vi "Engr_interface.vi"() -> ()   [LabVIEW 2016]
uses:
  Type_Defs/Digital_Out.ctl
  Type_Defs/Digital_In_1.ctl
  Type_Defs/Analog_In.ctl
  <vilib>/httpClient/ClientHandle.ctl
  msg7171_linux.llb/send single message.vi
  <vilib>/httpClient/POSTBuffer.vi
  <vilib>/httpClient/LabVIEWHTTPClient.lvlib
panel:
  out "Analog in":T1
  in  "LN2 Platen":u16(slide) max=4095 step=1 scale=0.0..4095.0
  in  "LN2 Shroud":u16(slide) max=4095 step=1 scale=0.0..4095.0
  out "Digi_In_1":T2
  in  "Digi_Out":T3
  in  "Regen Standby Mode SP":u8 max=1 step=1
  in  "Regen Repurge Time SP":u16=5 max=9999 step=1
  in  "Pumps per Compressor SP":u8=1 min=1 max=3 step=1
  in  "Regen Rough Interlock SP":u8=1 max=1 step=1
  in  "Regen Restart Temp SP":u8 max=80 step=1
  in  "Regen Rt of Rise Cycles SP":u8=50 max=200 step=1
  in  "Regen Rate of Rise SP":u8=10 min=1 max=100 step=1
  in  "Regen Rough to Press SP":u8=100 min=25 max=200 step=1
  in  "Regen Repurge Cycles SP":u8=50 max=200 step=1
  in  "Regen Ext Purge Time SP":u16 max=9990 step=1
  in  "MCC_2sgTempCtl":u16 max=320 step=1
  out "MCC_1sgTempCtll V":string
  out "MCC_2sgTempCtl V":string
  out "Regen Restart Delay":string
  in  "1st Ctl type":u8(ring) items=["ExtHeat", "1st s ctl", "2nd sctl", "Dual"]
  out "MCC_RegenCycles":string
  out "CryoP OP Time":string
  out "MCC_Status":string
  in  "Log?":bool
  out "Resp":string
  out "MCC Pwr":bool
  out "MCC Error":bool
  out "MCC_TurnTcOn_V":string
  out "MCC_TurnRoughOn_V":string
  out "MCC_TurnPurgeOn_V":string
  in  "MCC_StartRegen_V":u8(ring) items=["Abort Regen", "Start Full", "Start Fast", "Exit Standby", "Warm&Stop"]
  out "MCC 2nd stage Temp":string
  out "1st stage Temp":string
  out "MCCget_Ver_V":string
  out "MCC_RoughInterlock_V":string
  out "MCC_RegenSeq":string
  out "Regen Standby Mode":string
  out "Regen Repurge Time":string
  out "Pumps per Compressor":string
  out "Regen Rough Interlock":string
  out "Regen Restart Temp":string
  out "Regen Rt of Rise Cycles":string
  out "Regen Rate of Rise":string
  out "Regen Rough to Press":string
  out "Regen Repurge Cycles":string
  out "Regen Ext Purge Time":string
  in  "Regen Restart Delay SP":u16 max=59994 step=1
  out "DutyCycle":string
  out "MCC_TCpres":string
  in  "Get MCC":bool
  out "MCC_RegenTime":string
  in  "MCC_clearRoughInterlock":bool
  out "MCC_RegenError":string
  in  "MCC_StartRegen":bool
  in  "MCC_TurnTcOn":bool
  in  "MCC_OpenRoughGateValve":bool
  in  "MCC_OpenPurgeValve":bool
  in  "MCC_TurnPumpOn":bool
  in  "MCC_1sgTempCtl":u16 max=320 step=1
  in  "Params":bool
  in  "Get DIO":bool=TRUE
  in  "Get PG":bool
  out "x/y":T4 {"Rouffing Pump" format="%#_6e"; "Chamber Pressure" format="%#_6e"; "Cryo Pump" format="%#_6e"}
  in  "exit":bool
  out "Waveform Chart":waveform(dbl)[](graph)=[{"t0"=timestamp(3580757854.087 s since 1904-01-01), "dt"=1.0, "Y"=[750.0616827041697]}, {"t0"=timestamp(3580757854.087 s since 1904-01-01), "dt"=1.0, "Y"=[750.0616827041697]}, {"t0"=timestamp(3580757854.087 s since 1904-01-01), "dt"=1.0, "Y"=[750.0616827041697]}]
  out "MCC_PumpState":string
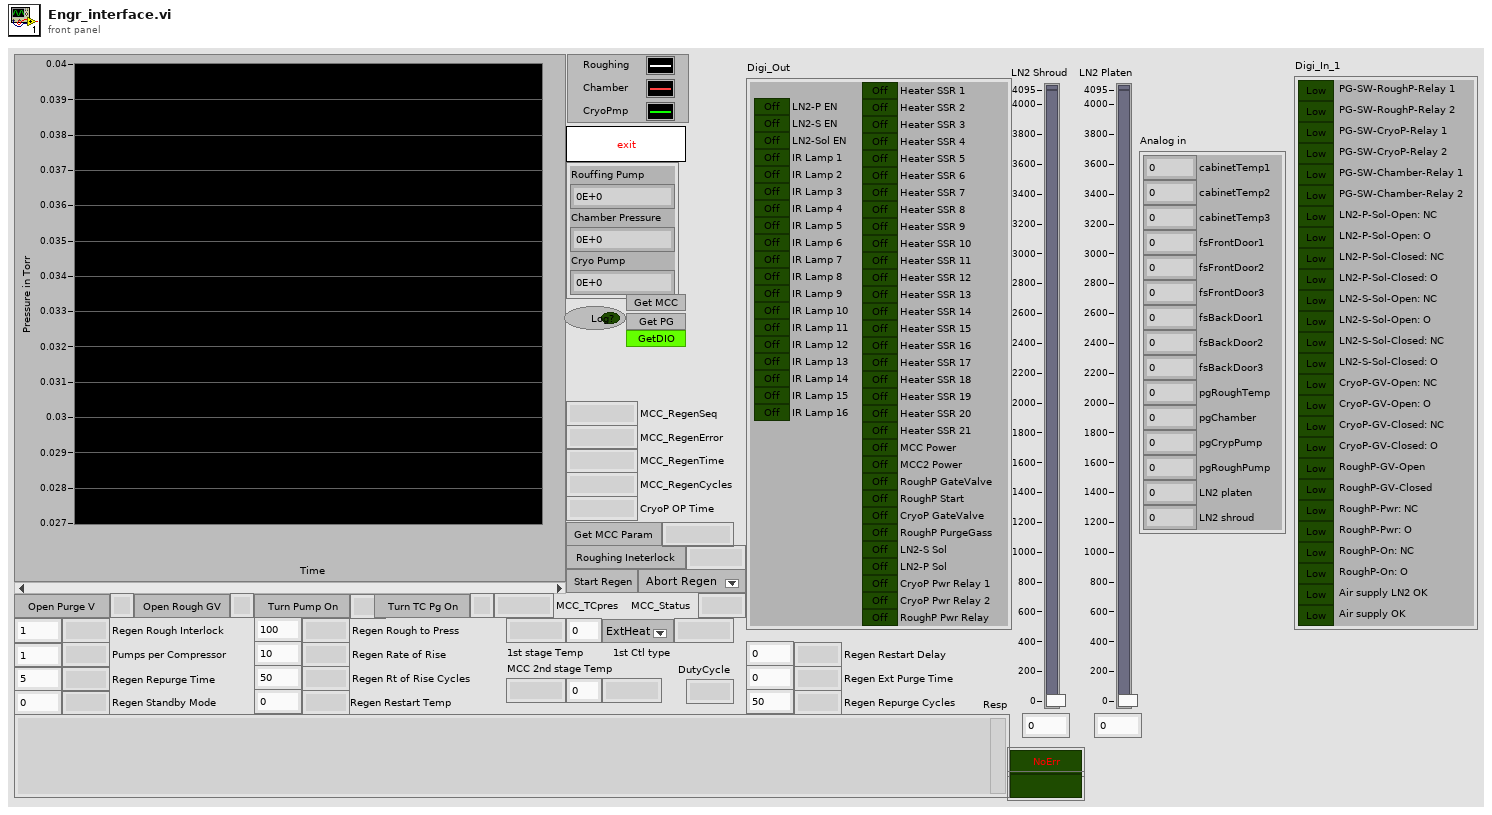
[diagram p1: front panel]
types:
  T1 = typedef "Analog_In.ctl" = cluster{"cabinetTemp1":u16, "cabinetTemp2":u16, "cabinetTemp3":u16, "fsFrontDoor1":u16, "fsFrontDoor2":u16, "fsFrontDoor3":u16, "fsBackDoor1":u16, "fsBackDoor2":u16, "fsBackDoor3":u16, "pgRoughTemp":u16, "pgChamber":u16, "pgCrypPump":u16, "pgRoughPump":u16, "LN2 platen":u16, "LN2 shroud":u16}
  T2 = typedef "Digital_In_1.ctl" = cluster{"PG-SW-RoughP-Relay 1":bool, "PG-SW-RoughP-Relay 2":bool, "PG-SW-CryoP-Relay 1":bool, "PG-SW-CryoP-Relay 2":bool, "PG-SW-Chamber-Relay 1":bool, "PG-SW-Chamber-Relay 2":bool, "LN2-P-Sol-Open: NC":bool, "LN2-P-Sol-Open: O":bool, "LN2-P-Sol-Closed: NC":bool, "LN2-P-Sol-Closed: O":bool, "LN2-S-Sol-Open: NC":bool, "LN2-S-Sol-Open: O":bool, "LN2-S-Sol-Closed: NC":bool, "LN2-S-Sol-Closed: O":bool, "CryoP-GV-Open: NC":bool, "CryoP-GV-Open: O":bool, "CryoP-GV-Closed: NC":bool, "CryoP-GV-Closed: O":bool, "RoughP-GV-Open":bool, "RoughP-GV-Closed":bool, "RoughP-Pwr: NC":bool, "RoughP-Pwr: O":bool, "RoughP-On: NC":bool, "RoughP-On: O":bool, "Air supply LN2 OK":bool, "Air supply OK":bool}
  T3 = typedef "Digital_Out.ctl" = cluster{"LN2-P EN":bool, "LN2-S EN":bool, "LN2-Sol EN":bool, "IR Lamp 1":bool, "IR Lamp 2":bool, "IR Lamp 3":bool, "IR Lamp 4":bool, "IR Lamp 5":bool, "IR Lamp 6":bool, "IR Lamp 7":bool, "IR Lamp 8":bool, "IR Lamp 9":bool, "IR Lamp 10":bool, "IR Lamp 11":bool, "IR Lamp 12":bool, "IR Lamp 13":bool, "IR Lamp 14":bool, "IR Lamp 15":bool, "IR Lamp 16":bool, "Heater SSR 1":bool, "Heater SSR 2":bool, "Heater SSR 3":bool, "Heater SSR 4":bool, "Heater SSR 5":bool, "Heater SSR 6":bool, "Heater SSR 7":bool, "Heater SSR 8":bool, "Heater SSR 9":bool, "Heater SSR 10":bool, "Heater SSR 11":bool, "Heater SSR 12":bool, "Heater SSR 13":bool, "Heater SSR 14":bool, "Heater SSR 15":bool, "Heater SSR 16":bool, "Heater SSR 17":bool, "Heater SSR 18":bool, "Heater SSR 19":bool, "Heater SSR 20":bool, "Heater SSR 21":bool, "MCC Power":bool, "MCC2 Power":bool, "RoughP GateValve":bool, "RoughP Start":bool, "CryoP GateValve":bool, "RoughP PurgeGass":bool, "LN2-S Sol":bool, "LN2-P Sol":bool, "CryoP Pwr Relay 1":bool, "CryoP Pwr Relay 2":bool, "RoughP Pwr Relay":bool}
  T4 = cluster{"Rouffing Pump":dbl, "Chamber Pressure":dbl, "Cryo Pump":dbl}
  T5 = typedef "LabVIEWHTTPClient.lvlib/ClientHandle.ctl" = refnum<k1>
  T6 = cluster{"go":bool, "Http session":T5, "URL prefex":string}
  T7 = cluster{"Addr":i32[], "Kind":string[], "Pressure":dbl[], "Sw1 SP":dbl[], "Sw2 SP":dbl[]}
  T8 = cluster{"Error":bool, "PowerFailure":bool, "Data":string}
  T9 = cluster{"Status":string, "TcPressure":string, "TempStage1":string, "TempStage2":string, "Duty Cycle":string, "RegenStep":string, "RegenError":string, "CryoPumpRdyState":string}
  T10 = cluster{"MCCVersion":string, "ElapsedTime":string, "FirstStageTempCTL":string, "PurgeValveState":string, "RegenCycles":string, "RegenParam_0":string, "RegenParam_1":string, "RegenParam_2":string, "RegenParam_3":string, "RegenParam_4":string, "RegenParam_5":string, "RegenParam_6":string, "RegenParam_A":string, "RegenParam_C":string, "RegenParam_G":string, "RegenParam_z":string, "RegenTime":string, "RoughingValveState":string, "RoughingInterlock":string, "SecondStageTempCTL":string, "TcPressureState":string}
  T11 = cluster{"event":string, "event":string, "JSON string":string}
  T12 = cluster{"event":string, "event":string, "event":string}
  T13 = cluster{"Pressure[0]":dbl, "Pressure[1]":dbl, "Pressure[2]":dbl}
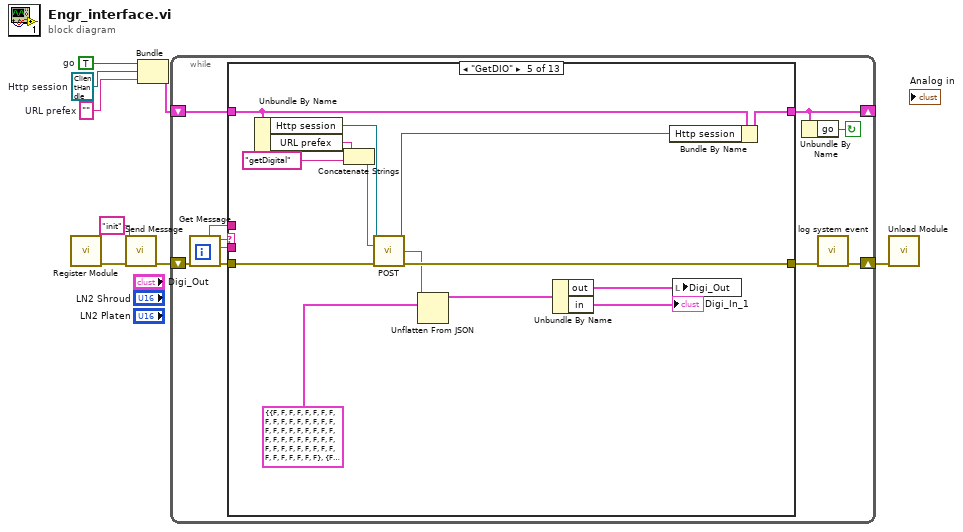
[diagram p0: block diagram]
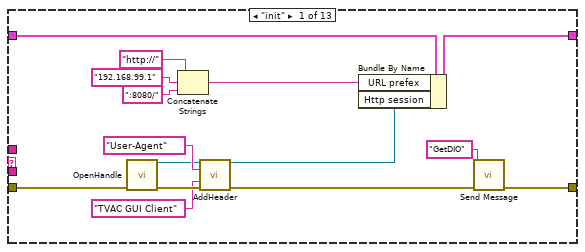
[diagram p2: hidden frame]
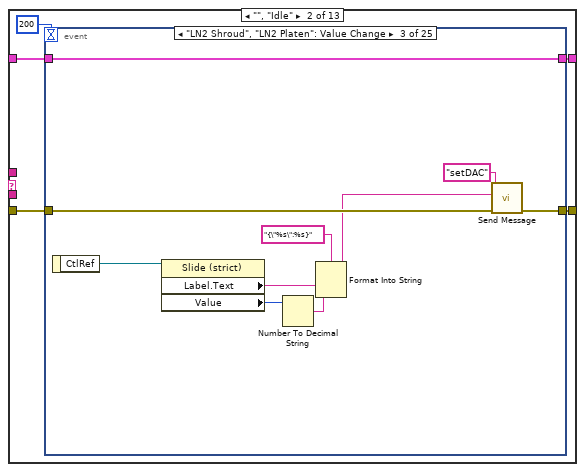
[diagram p3: hidden frame]
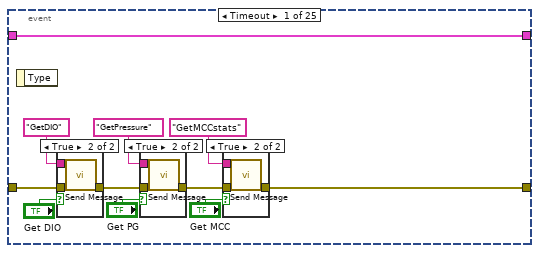
[diagram p4: hidden frame]
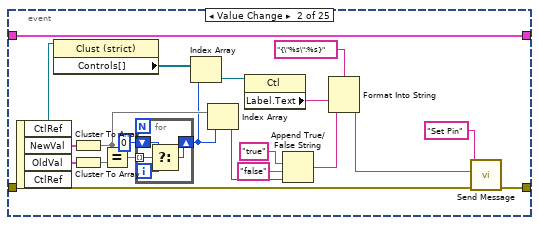
[diagram p8: hidden frame]
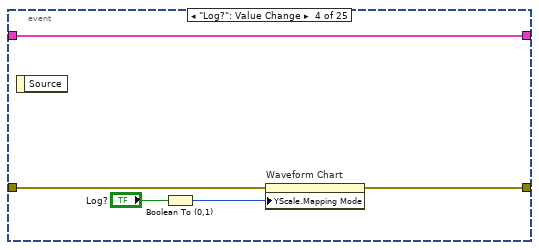
[diagram p9: hidden frame]
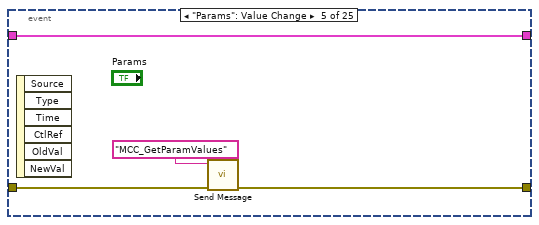
[diagram p10: hidden frame]
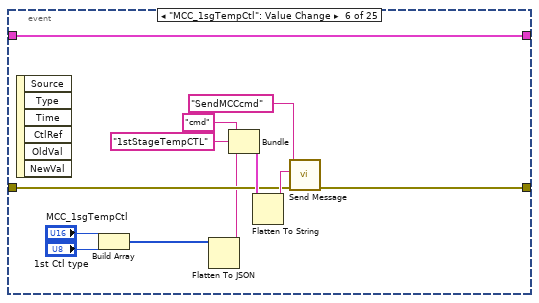
[diagram p11: hidden frame]
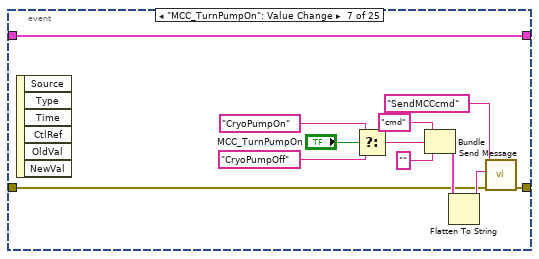
[diagram p12: hidden frame]
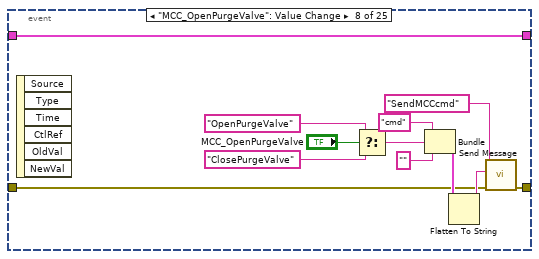
[diagram p13: hidden frame]
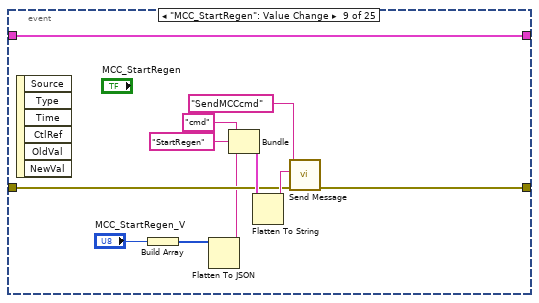
[diagram p14: hidden frame]
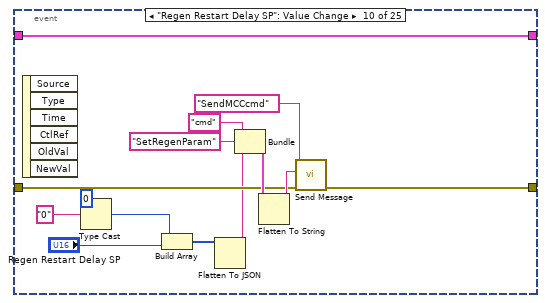
[diagram p15: hidden frame]
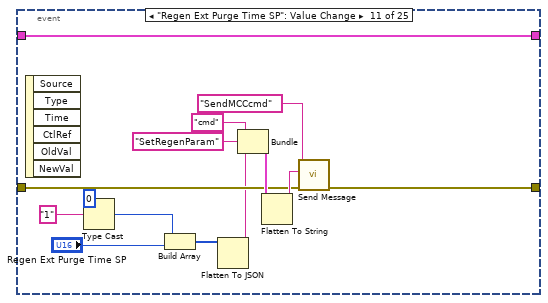
[diagram p16: hidden frame]
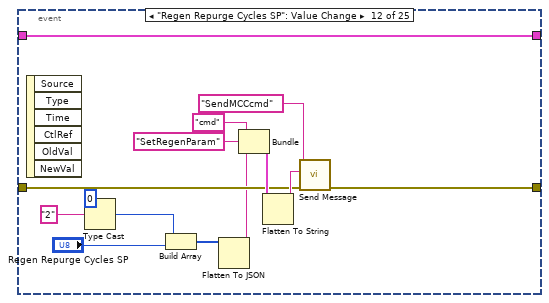
[diagram p17: hidden frame]
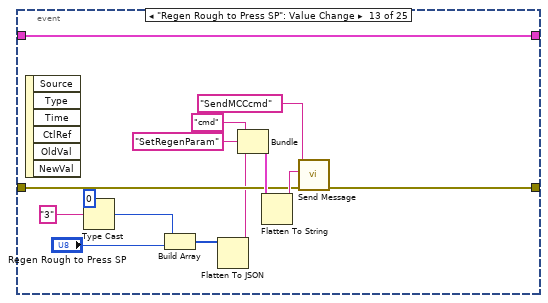
[diagram p18: hidden frame]
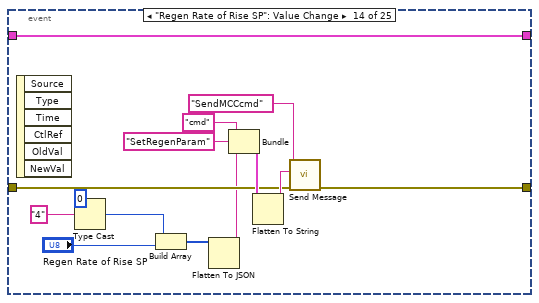
[diagram p19: hidden frame]
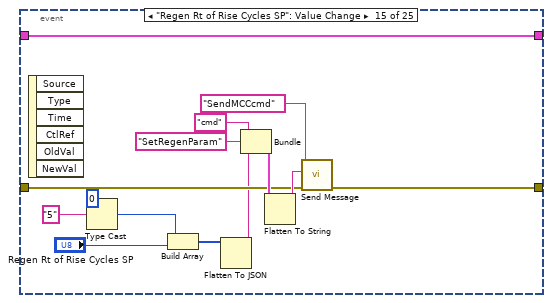
[diagram p20: hidden frame]
diagram:
  w4 = ""  # URL prefex
  w5 = T5 refnum  # Http session
  w6 = TRUE  # go
  n1 = call "Register Module.vi"() -> ("error out"=w2:errorcluster)  [unwired: 10 in, 1 out]
  n2 = call-poly "Send Message.vi"("error in (no error)"=w2, "event"="init") -> ("error out"=w1:errorcluster)  [unwired: 9 in]
  n3 = Bundle("go"=w6, "Http session"=w5, "URL prefex"=w4) -> (w8:T6)  [unwired: 1 in]
  n4 = while {
    shift-left: w8 -> [w15]
    shift-right: [w12] -> _
    shift-right: [w10] -> w7
    shift-left: w1 -> [w18]
    stop <- w11 continue-if-true
    n5 = call "Get Message.vi"("error in (no error)"=w18) -> ("error out"=w16:errorcluster, "event buffer"=w17:string, "event"=w14:string, "source"=w13:string)  [unwired: 7 in]
    n6 = case shown="\"GetDIO\"" w14 {
      selector: w14 -> [_ _ w360 _ _ _ _ _ _ _ _ _ w540]
      tunnel: [w24 w35 w364 w386 w398 w418 w447 w456 w473 w504 w531 w537 w542] -> w12
      tunnel: w15 -> [w33 w34 w363 w385 w397 w416 w447 w456 w471 w504 w531 w532 w542]
      tunnel: w17 -> [_ _ w358 w382 _ _ _ _ w465 w502 w529 _ _]
      tunnel: w16 -> [w28 w36 w362 w384 w400 w420 w440 w449 w474 w505 w530 w535 w541]
      tunnel: w13 -> [_ _ _ _ _ _ _ _ _ _ _ _ w539]
      tunnel: [w20 w38 w361 w383 w399 w419 w439 w448 w459 w505 w530 w534 w538] -> w9
      frame "init" {
        n7 = call <vilib>:"OpenHandle.vi"("error in (no error)"=w28) -> ("client handle out"=w29:T5, "error out"=w32:errorcluster)  [unwired: 13 in]
        n8 = Concatenate Strings("http://" ("url"), "192.168.99.1" ("Address"), ":8080/" ("url")) -> (w23:string)
        n9 = call <vilib>:"AddHeader.vi"("client handle"=w29, "header"="User-Agent", "value"="TVAC GUI Client", "error in (no error)"=w32) -> ("client handle out"=w22:T5, "error out"=w21:errorcluster)  [unwired: 10 in]
        n10 = Bundle By Name(cluster=w33, "URL prefex"=w23, "Http session"=w22) -> (w24:T6)
        n11 = call-poly "Send Message.vi"("error in (no error)"=w21, "event"="GetDIO") -> ("error out"=w20:errorcluster)  [unwired: 9 in]
      }
      frame "", "Idle" {
        n12 = event shown="[2] \"LN2 Shroud\", \"LN2 Platen\": Value Change" {
          selector: _ -> [_ _ _ _ _ _ _ _ _ _ _ _ _ _ _ _ _ _ _ _ _ _ _ _ _]
          dyn-events: _ -> [_ _ _ _ _ _ _ _ _ _ _ _ _ _ _ _ _ _ _ _ _ _ _ _ _]
          timeout: 200 ("milliseconds to wait") -> [_ _ _ _ _ _ _ _ _ _ _ _ _ _ _ _ _ _ _ _ _ _ _ _ _]
          tunnel: w36 -> [w48 w77 w94 w100 w104 w111 w123 w135 w146 w160 w174 w188 w202 w216 w230 w244 w258 w272 w286 w300 w312 w322 w332 w344 w354]
          tunnel: [w39 w76 w95 w99 w103 w110 w122 w134 w145 w159 w173 w187 w201 w215 w229 w243 w257 w271 w285 w299 w311 w321 w331 w343 w353] -> w38
          tunnel: [w49 w82 w87 w101 w102 w112 w124 w136 w147 w161 w175 w189 w203 w217 w231 w245 w259 w273 w287 w301 w313 w323 w333 w345 w351] -> w35
          tunnel: w34 -> [w49 w82 w87 w101 w102 w112 w124 w136 w147 w161 w175 w189 w203 w217 w231 w245 w259 w273 w287 w301 w313 w323 w333 w345 w351]
          event Timeout {
            n13 = event-data() -> ()  [unwired: 1 in, 1 out]
            n14 = case shown="True" "Get DIO" {
              tunnel: w48 -> [w58 w61]
              tunnel: [w58 w60] -> w46
              tunnel: "GetDIO" ("event") -> [_ w59]
              frame False {
              }
              frame True {
                n15 = call-poly "Send Message.vi"("error in (no error)"=w61, "event"=w59) -> ("error out"=w60:errorcluster)  [unwired: 9 in]
              }
            }
            n16 = case shown="True" "Get PG" {
              tunnel: w46 -> [w54 w57]
              tunnel: [w54 w56] -> w40
              tunnel: "GetPressure" ("event") -> [_ w55]
              frame False {
              }
              frame True {
                n17 = call-poly "Send Message.vi"("error in (no error)"=w57, "event"=w55) -> ("error out"=w56:errorcluster)  [unwired: 9 in]
              }
            }
            n18 = case shown="True" "Get MCC" {
              tunnel: w40 -> [w50 w53]
              tunnel: [w50 w52] -> w39
              tunnel: "GetMCCstats" ("event") -> [_ w51]
              frame False {
              }
              frame True {
                n19 = call-poly "Send Message.vi"("error in (no error)"=w53, "event"=w51) -> ("error out"=w52:errorcluster)  [unwired: 9 in]
              }
            }
          }
          event Value Change {
            n20 = event-data() -> ("CtlRef"=w63:refnum<vi>, "NewVal"=w78:T3, "OldVal"=w81:T3)  [unwired: 1 in, 1 out]
            n21 = property class="Clust (strict)"(reference=w63) -> ("Controls[]"=w73:refnum<vi>[])  [unwired: 1 in, 2 out]
            n22 = Cluster To Array(cluster=w78) -> (array=w74:bool[])
            n23 = Cluster To Array(cluster=w81) -> (array=w75:bool[])
            n24 = Equal?(x=w74, y=w75) -> (x = y?=w80:bool[])
            n25 = for {
              tunnel: w80 -> [w86] mode=indexing
              shift-right: [w85] -> w72
              shift-left: 0 -> [w84]
              i -> [w83]
              n26 = Select(t=w84, s=w86, f=w83) -> (s? t:f=w85:i32)
            }
            n27 = Index Array(array=w73, index=w72) -> (element=w71:refnum<vi>)
            n28 = Index Array(array=w74, index=w72) -> (element=w69:bool)
            n29 = property class="Ctl"(reference=w71) -> ("Label.Text"=w66:string)  [unwired: 1 in, 2 out]
            n30 = Append True/False String(1:w69, 2:"false" ("false string"), 3:"true" ("true string")) -> (0:w64:string)  [unwired: 1 in]
            n31 = Format Into String(format string="{\"%s\":%s}" ("string"), w66, w64) -> (resulting string=w62:string)  [unwired: 2 in, 1 out]
            n32 = call-poly "Send Message.vi"("error in (no error)"=w77, "event buffer"=w62, "event"="Set Pin") -> ("error out"=w76:errorcluster)  [unwired: 8 in]
          }
          event "LN2 Shroud", "LN2 Platen": Value Change {
            n33 = event-data() -> ("CtlRef"=w93:refnum<vi>)  [unwired: 1 in]
            n34 = property class="Slide (strict)"(reference=w93) -> ("Label.Text"=w91:string, "Value"=w90:u16)  [unwired: 1 in, 2 out]
            n35 = Number To Decimal String(number=w90) -> (decimal integer string=w89:string)  [unwired: 1 in]
            n36 = Format Into String(format string="{\"%s\":%s}" ("string"), w91, w89) -> (resulting string=w88:string)  [unwired: 2 in, 1 out]
            n37 = call-poly "Send Message.vi"("error in (no error)"=w94, "event buffer"=w88, "event"="setDAC") -> ("error out"=w95:errorcluster)  [unwired: 8 in]
          }
          event "Log?": Value Change {
            n38 = event-data() -> ()  [unwired: 1 in, 1 out]
            n39 = Boolean To (0,1)(Boolean="Log?") -> (0, 1=w98:i16)
            n40 = property on="Waveform Chart" class="WFChart (strict)"(error in=w100, "YScale.Mapping Mode"=w98) -> (error out=w99:errorcluster)  [unwired: 1 in, 1 out]
          }
          event "Params": Value Change {
            n41 = event-data() -> ()  [unwired: 1 in, 6 out]
            n42 = call-poly "Send Message.vi"("error in (no error)"=w104, "event"="MCC_GetParamValues") -> ("error out"=w103:errorcluster)  [unwired: 9 in]
          }
          event "MCC_1sgTempCtl": Value Change {
            n43 = event-data() -> ()  [unwired: 1 in, 6 out]
            n44 = Build Array("MCC_1sgTempCtl", "1st Ctl type") -> (w107:u16[])
            n45 = Flatten To JSON(anything=w107) -> (JSON string=w106:string)  [unwired: 2 in, 1 out]
            n46 = Bundle("event"="cmd", "event"="1stStageTempCTL", "JSON string"=w106) -> (w115:T11)  [unwired: 1 in]
            n47 = Flatten To String(anything=w115) -> (data string=w116:string)  [unwired: 3 in, 2 out]
            n48 = call-poly "Send Message.vi"("error in (no error)"=w111, "event buffer"=w116, "event"="SendMCCcmd") -> ("error out"=w110:errorcluster)  [unwired: 8 in]
          }
          event "MCC_TurnPumpOn": Value Change {
            n49 = event-data() -> ()  [unwired: 1 in, 6 out]
            n50 = Select(t="CryoPumpOn" ("event"), s="MCC_TurnPumpOn", f="CryoPumpOff" ("event")) -> (s? t:f=w120:string)
            n51 = Bundle("event"="cmd", "event"=w120, "event"="") -> (w127:T12)  [unwired: 1 in]
            n52 = Flatten To String(anything=w127) -> (data string=w128:string)  [unwired: 3 in, 2 out]
            n53 = call-poly "Send Message.vi"("error in (no error)"=w123, "event buffer"=w128, "event"="SendMCCcmd") -> ("error out"=w122:errorcluster)  [unwired: 8 in]
          }
          event "MCC_OpenPurgeValve": Value Change {
            n54 = event-data() -> ()  [unwired: 1 in, 6 out]
            n55 = Select(t="OpenPurgeValve" ("event"), s="MCC_OpenPurgeValve", f="ClosePurgeValve" ("event")) -> (s? t:f=w132:string)
            n56 = Bundle("event"="cmd", "event"=w132, "event"="") -> (w139:T12)  [unwired: 1 in]
            n57 = Flatten To String(anything=w139) -> (data string=w140:string)  [unwired: 3 in, 2 out]
            n58 = call-poly "Send Message.vi"("error in (no error)"=w135, "event buffer"=w140, "event"="SendMCCcmd") -> ("error out"=w134:errorcluster)  [unwired: 8 in]
          }
          event "MCC_StartRegen": Value Change {
            n59 = event-data() -> ()  [unwired: 1 in, 6 out]
            n60 = Build Array("MCC_StartRegen_V") -> (w143:u8[])
            n61 = Flatten To JSON(anything=w143) -> (JSON string=w144:string)  [unwired: 2 in, 1 out]
            n62 = Bundle("event"="cmd", "event"="StartRegen", "JSON string"=w144) -> (w150:T11)  [unwired: 1 in]
            n63 = Flatten To String(anything=w150) -> (data string=w151:string)  [unwired: 3 in, 2 out]
            n64 = call-poly "Send Message.vi"("error in (no error)"=w146, "event buffer"=w151, "event"="SendMCCcmd") -> ("error out"=w145:errorcluster)  [unwired: 8 in]
          }
          event "Regen Restart Delay SP": Value Change {
            n65 = event-data() -> ()  [unwired: 1 in, 6 out]
            n66 = Type Cast(type=u8 0 ("unsigned 8bit integer"), x="0") -> (*(type *) &x=w154:u8)
            n67 = Build Array(w154, "Regen Restart Delay SP") -> (w158:u16[])
            n68 = Flatten To JSON(anything=w158) -> (JSON string=w157:string)  [unwired: 2 in, 1 out]
            n69 = Bundle("event"="cmd", "event"="SetRegenParam", "JSON string"=w157) -> (w164:T11)  [unwired: 1 in]
            n70 = Flatten To String(anything=w164) -> (data string=w165:string)  [unwired: 3 in, 2 out]
            n71 = call-poly "Send Message.vi"("error in (no error)"=w160, "event buffer"=w165, "event"="SendMCCcmd") -> ("error out"=w159:errorcluster)  [unwired: 8 in]
          }
          event "Regen Ext Purge Time SP": Value Change {
            n72 = event-data() -> ()  [unwired: 1 in, 6 out]
            n73 = Type Cast(type=u8 0 ("unsigned 8bit integer"), x="1") -> (*(type *) &x=w168:u8)
            n74 = Build Array(w168, "Regen Ext Purge Time SP") -> (w172:u16[])
            n75 = Flatten To JSON(anything=w172) -> (JSON string=w171:string)  [unwired: 2 in, 1 out]
            n76 = Bundle("event"="cmd", "event"="SetRegenParam", "JSON string"=w171) -> (w178:T11)  [unwired: 1 in]
            n77 = Flatten To String(anything=w178) -> (data string=w179:string)  [unwired: 3 in, 2 out]
            n78 = call-poly "Send Message.vi"("error in (no error)"=w174, "event buffer"=w179, "event"="SendMCCcmd") -> ("error out"=w173:errorcluster)  [unwired: 8 in]
          }
          event "Regen Repurge Cycles SP": Value Change {
            n79 = event-data() -> ()  [unwired: 1 in, 6 out]
            n80 = Type Cast(type=u8 0 ("unsigned 8bit integer"), x="2") -> (*(type *) &x=w182:u8)
            n81 = Build Array(w182, "Regen Repurge Cycles SP") -> (w186:u8[])
            n82 = Flatten To JSON(anything=w186) -> (JSON string=w185:string)  [unwired: 2 in, 1 out]
            n83 = Bundle("event"="cmd", "event"="SetRegenParam", "JSON string"=w185) -> (w192:T11)  [unwired: 1 in]
            n84 = Flatten To String(anything=w192) -> (data string=w193:string)  [unwired: 3 in, 2 out]
            n85 = call-poly "Send Message.vi"("error in (no error)"=w188, "event buffer"=w193, "event"="SendMCCcmd") -> ("error out"=w187:errorcluster)  [unwired: 8 in]
          }
          event "Regen Rough to Press SP": Value Change {
            n86 = event-data() -> ()  [unwired: 1 in, 6 out]
            n87 = Type Cast(type=u8 0 ("unsigned 8bit integer"), x="3") -> (*(type *) &x=w196:u8)
            n88 = Build Array(w196, "Regen Rough to Press SP") -> (w200:u8[])
            n89 = Flatten To JSON(anything=w200) -> (JSON string=w199:string)  [unwired: 2 in, 1 out]
            n90 = Bundle("event"="cmd", "event"="SetRegenParam", "JSON string"=w199) -> (w206:T11)  [unwired: 1 in]
            n91 = Flatten To String(anything=w206) -> (data string=w207:string)  [unwired: 3 in, 2 out]
            n92 = call-poly "Send Message.vi"("error in (no error)"=w202, "event buffer"=w207, "event"="SendMCCcmd") -> ("error out"=w201:errorcluster)  [unwired: 8 in]
          }
          event "Regen Rate of Rise SP": Value Change {
            n93 = event-data() -> ()  [unwired: 1 in, 6 out]
            n94 = Type Cast(type=u8 0 ("unsigned 8bit integer"), x="4") -> (*(type *) &x=w210:u8)
            n95 = Build Array(w210, "Regen Rate of Rise SP") -> (w214:u8[])
            n96 = Flatten To JSON(anything=w214) -> (JSON string=w213:string)  [unwired: 2 in, 1 out]
            n97 = Bundle("event"="cmd", "event"="SetRegenParam", "JSON string"=w213) -> (w220:T11)  [unwired: 1 in]
            n98 = Flatten To String(anything=w220) -> (data string=w221:string)  [unwired: 3 in, 2 out]
            n99 = call-poly "Send Message.vi"("error in (no error)"=w216, "event buffer"=w221, "event"="SendMCCcmd") -> ("error out"=w215:errorcluster)  [unwired: 8 in]
          }
          event "Regen Rt of Rise Cycles SP": Value Change {
            n100 = event-data() -> ()  [unwired: 1 in, 6 out]
            n101 = Type Cast(type=u8 0 ("unsigned 8bit integer"), x="5") -> (*(type *) &x=w224:u8)
            n102 = Build Array(w224, "Regen Rt of Rise Cycles SP") -> (w228:u8[])
            n103 = Flatten To JSON(anything=w228) -> (JSON string=w227:string)  [unwired: 2 in, 1 out]
            n104 = Bundle("event"="cmd", "event"="SetRegenParam", "JSON string"=w227) -> (w234:T11)  [unwired: 1 in]
            n105 = Flatten To String(anything=w234) -> (data string=w235:string)  [unwired: 3 in, 2 out]
            n106 = call-poly "Send Message.vi"("error in (no error)"=w230, "event buffer"=w235, "event"="SendMCCcmd") -> ("error out"=w229:errorcluster)  [unwired: 8 in]
          }
          event "Regen Restart Temp SP": Value Change {
            n107 = event-data() -> ()  [unwired: 1 in, 6 out]
            n108 = Type Cast(type=u8 0 ("unsigned 8bit integer"), x="6") -> (*(type *) &x=w238:u8)
            n109 = Build Array(w238, "Regen Restart Temp SP") -> (w242:u8[])
            n110 = Flatten To JSON(anything=w242) -> (JSON string=w241:string)  [unwired: 2 in, 1 out]
            n111 = Bundle("event"="cmd", "event"="SetRegenParam", "JSON string"=w241) -> (w248:T11)  [unwired: 1 in]
            n112 = Flatten To String(anything=w248) -> (data string=w249:string)  [unwired: 3 in, 2 out]
            n113 = call-poly "Send Message.vi"("error in (no error)"=w244, "event buffer"=w249, "event"="SendMCCcmd") -> ("error out"=w243:errorcluster)  [unwired: 8 in]
          }
          event "Regen Rough Interlock SP": Value Change {
            n114 = event-data() -> ()  [unwired: 1 in, 6 out]
            n115 = Type Cast(type=u8 0 ("unsigned 8bit integer"), x="A") -> (*(type *) &x=w252:u8)
            n116 = Build Array(w252, "Regen Rough Interlock SP") -> (w256:u8[])
            n117 = Flatten To JSON(anything=w256) -> (JSON string=w255:string)  [unwired: 2 in, 1 out]
            n118 = Bundle("event"="cmd", "event"="SetRegenParam", "JSON string"=w255) -> (w262:T11)  [unwired: 1 in]
            n119 = Flatten To String(anything=w262) -> (data string=w263:string)  [unwired: 3 in, 2 out]
            n120 = call-poly "Send Message.vi"("error in (no error)"=w258, "event buffer"=w263, "event"="SendMCCcmd") -> ("error out"=w257:errorcluster)  [unwired: 8 in]
          }
          event "Pumps per Compressor SP": Value Change {
            n121 = event-data() -> ()  [unwired: 1 in, 6 out]
            n122 = Type Cast(type=u8 0 ("unsigned 8bit integer"), x="C") -> (*(type *) &x=w266:u8)
            n123 = Build Array(w266, "Pumps per Compressor SP") -> (w270:u8[])
            n124 = Flatten To JSON(anything=w270) -> (JSON string=w269:string)  [unwired: 2 in, 1 out]
            n125 = Bundle("event"="cmd", "event"="SetRegenParam", "JSON string"=w269) -> (w276:T11)  [unwired: 1 in]
            n126 = Flatten To String(anything=w276) -> (data string=w277:string)  [unwired: 3 in, 2 out]
            n127 = call-poly "Send Message.vi"("error in (no error)"=w272, "event buffer"=w277, "event"="SendMCCcmd") -> ("error out"=w271:errorcluster)  [unwired: 8 in]
          }
          event "Regen Repurge Time SP": Value Change {
            n128 = event-data() -> ()  [unwired: 1 in, 6 out]
            n129 = Type Cast(type=u8 0 ("unsigned 8bit integer"), x="G") -> (*(type *) &x=w280:u8)
            n130 = Build Array(w280, "Regen Repurge Time SP") -> (w284:u16[])
            n131 = Flatten To JSON(anything=w284) -> (JSON string=w283:string)  [unwired: 2 in, 1 out]
            n132 = Bundle("event"="cmd", "event"="SetRegenParam", "JSON string"=w283) -> (w290:T11)  [unwired: 1 in]
            n133 = Flatten To String(anything=w290) -> (data string=w291:string)  [unwired: 3 in, 2 out]
            n134 = call-poly "Send Message.vi"("error in (no error)"=w286, "event buffer"=w291, "event"="SendMCCcmd") -> ("error out"=w285:errorcluster)  [unwired: 8 in]
          }
          event "Regen Standby Mode SP": Value Change {
            n135 = event-data() -> ()  [unwired: 1 in, 6 out]
            n136 = Type Cast(type=u8 0 ("unsigned 8bit integer"), x="z") -> (*(type *) &x=w294:u8)
            n137 = Build Array(w294, "Regen Standby Mode SP") -> (w298:u8[])
            n138 = Flatten To JSON(anything=w298) -> (JSON string=w297:string)  [unwired: 2 in, 1 out]
            n139 = Bundle("event"="cmd", "event"="SetRegenParam", "JSON string"=w297) -> (w304:T11)  [unwired: 1 in]
            n140 = Flatten To String(anything=w304) -> (data string=w305:string)  [unwired: 3 in, 2 out]
            n141 = call-poly "Send Message.vi"("error in (no error)"=w300, "event buffer"=w305, "event"="SendMCCcmd") -> ("error out"=w299:errorcluster)  [unwired: 8 in]
          }
          event "MCC_OpenRoughGateValve": Value Change {
            n142 = event-data() -> ()  [unwired: 1 in, 6 out]
            n143 = Select(t="OpenRoughValve" ("event"), s="MCC_OpenRoughGateValve", f="CloseRoughValve" ("event")) -> (s? t:f=w309:string)
            n144 = Bundle("event"="cmd", "event"=w309, "event"="") -> (w316:T12)  [unwired: 1 in]
            n145 = Flatten To String(anything=w316) -> (data string=w317:string)  [unwired: 3 in, 2 out]
            n146 = call-poly "Send Message.vi"("error in (no error)"=w312, "event buffer"=w317, "event"="SendMCCcmd") -> ("error out"=w311:errorcluster)  [unwired: 8 in]
          }
          event "MCC_clearRoughInterlock": Value Change {
            n147 = event-data() -> ()  [unwired: 1 in, 6 out]
            n148 = Bundle("event"="cmd", "event"="ClearInterlock", "event"="") -> (w325:T12)  [unwired: 1 in]
            n149 = Flatten To String(anything=w325) -> (data string=w326:string)  [unwired: 3 in, 2 out]
            n150 = call-poly "Send Message.vi"("error in (no error)"=w322, "event buffer"=w326, "event"="SendMCCcmd") -> ("error out"=w321:errorcluster)  [unwired: 8 in]
          }
          event "MCC_2sgTempCtl": Value Change {
            n151 = event-data() -> ()  [unwired: 1 in, 6 out]
            n152 = Build Array("MCC_2sgTempCtl") -> (w328:u16[])
            n153 = Flatten To JSON(anything=w328) -> (JSON string=w330:string)  [unwired: 2 in, 1 out]
            n154 = Bundle("event"="cmd", "event"="2ndStageTempCTL", "JSON string"=w330) -> (w336:T11)  [unwired: 1 in]
            n155 = Flatten To String(anything=w336) -> (data string=w337:string)  [unwired: 3 in, 2 out]
            n156 = call-poly "Send Message.vi"("error in (no error)"=w332, "event buffer"=w337, "event"="SendMCCcmd") -> ("error out"=w331:errorcluster)  [unwired: 8 in]
          }
          event "MCC_TurnTcOn": Value Change {
            n157 = event-data() -> ()  [unwired: 1 in, 6 out]
            n158 = Select(t="TurnTcPresOn" ("event"), s="MCC_TurnTcOn", f="TurnTcPresOff" ("event")) -> (s? t:f=w341:string)
            n159 = Bundle("event"="cmd", "event"=w341, "event"="") -> (w348:T12)  [unwired: 1 in]
            n160 = Flatten To String(anything=w348) -> (data string=w349:string)  [unwired: 3 in, 2 out]
            n161 = call-poly "Send Message.vi"("error in (no error)"=w344, "event buffer"=w349, "event"="SendMCCcmd") -> ("error out"=w343:errorcluster)  [unwired: 8 in]
          }
          event "exit": Value Change {
            n162 = event-data() -> ()  [unwired: 1 in, 1 out]
            n163 = call "Deliver Message.vi"("error in (no error)"=w354, "event"="exit") -> ("error out"=w353:errorcluster)  [unwired: 9 in]
          }
        }
      }
      frame "Set Pin" {
        (unwired) "{\"RoughP Start\":true}" ("string")
        n164 = Unbundle By Name(w363) -> ("Http session"=w368:T5, "URL prefex"=w366:string)
        n165 = Concatenate Strings(w366, "setDigital" ("url")) -> (w367:string)
        n166 = call-poly <vilib>:"POST.vi"("client handle"=w368, "url"=w367, "buffer"=w358, "error in (no error)"=w362) -> ("client handle out"=w369:T5, "error out"=w359:errorcluster)  [unwired: 8 in, 2 out]
        n167 = Build Array(0) -> (w356:i32[])
        n168 = case shown="False" FALSE {
          tunnel: [w370 w381] -> w361
          tunnel: w360 -> [_ w380]
          tunnel: w359 -> [w370 w379]
          tunnel: w356 -> [_ w376]
          frame False {
          }
          frame True {
            n169 = Replace Array Subset(array=w376, new element=0 ("new element/subarray"), index=2) -> (w372:i32[])
            n170 = call-poly "Send Message.vi"("error in (no error)"=w379, "event"="GetDIO") -> ("error out"=w378:errorcluster)  [unwired: 9 in]
            n171 = Flatten To JSON(anything=w372) -> (JSON string=w373:string)  [unwired: 2 in, 1 out]
            n172 = Wait (ms)(milliseconds to wait=u32 50) -> ()  [unwired: 1 out]
            n173 = call-poly "Send Message.vi"("error in (no error)"=w378, "event buffer"=w373, "event"=w380) -> ("error out"=w381:errorcluster)  [unwired: 8 in]
          }
        }
        n174 = Bundle By Name(cluster=w363, "Http session"=w369) -> (w364:T6)
      }
      frame "setDAC" {
        n175 = Unbundle By Name(w385) -> ("Http session"=w390:T5, "URL prefex"=w388:string)
        n176 = Concatenate Strings(w388, "setAnalog" ("url")) -> (w389:string)
        n177 = call-poly <vilib>:"POST.vi"("client handle"=w390, "url"=w389, "buffer"=w382, "error in (no error)"=w384) -> ("client handle out"=w391:T5, "error out"=w383:errorcluster)  [unwired: 8 in, 2 out]
        n178 = Bundle By Name(cluster=w385, "Http session"=w391) -> (w386:T6)
      }
      frame "GetDIO" {
        n179 = Unbundle By Name(w397) -> ("Http session"=w404:T5, "URL prefex"=w402:string)
        n180 = Concatenate Strings(w402, "getDigital" ("url")) -> (w403:string)
        n181 = call-poly <vilib>:"POST.vi"("client handle"=w404, "url"=w403, "error in (no error)"=w400) -> ("client handle out"=w405:T5, "body"=w396:string, "error out"=w399:errorcluster)  [unwired: 9 in, 1 out]
        n182 = Unflatten From JSON(JSON string=w396, type and defaults=cluster{"out":T3, "in":T2} {"out"={"LN2-P EN"=FALSE, "LN2-S EN"=FALSE, "LN2-Sol EN"=FALSE, "IR Lamp 1"=FALSE, "IR Lamp 2"=FALSE, "IR Lamp 3"=FALSE, "IR Lamp 4"=FALSE, "IR Lamp 5"=FALSE, "IR Lamp 6"=FALSE, "IR Lamp 7"=FALSE, "IR Lamp 8"=FALSE, "IR Lamp 9"=FALSE, "IR Lamp 10"=FALSE, "IR Lamp 11"=FALSE, "IR Lamp 12"=FALSE, "IR Lamp 13"=FALSE, "IR Lamp 14"=FALSE, "IR Lamp 15"=FALSE, "IR Lamp 16"=FALSE, "Heater SSR 1"=FALSE, "Heater SSR 2"=FALSE, "Heater SSR 3"=FALSE, "Heater SSR 4"=FALSE, "Heater SSR 5"=FALSE, "Heater SSR 6"=FALSE, "Heater SSR 7"=FALSE, "Heater SSR 8"=FALSE, "Heater SSR 9"=FALSE, "Heater SSR 10"=FALSE, "Heater SSR 11"=FALSE, "Heater SSR 12"=FALSE, "Heater SSR 13"=FALSE, "Heater SSR 14"=FALSE, "Heater SSR 15"=FALSE, "Heater SSR 16"=FALSE, "Heater SSR 17"=FALSE, "Heater SSR 18"=FALSE, "Heater SSR 19"=FALSE, "Heater SSR 20"=FALSE, "Heater SSR 21"=FALSE, "MCC Power"=FALSE, "MCC2 Power"=FALSE, "RoughP GateValve"=FALSE, "RoughP Start"=FALSE, "CryoP GateValve"=FALSE, "RoughP PurgeGass"=FALSE, "LN2-S Sol"=FALSE, "LN2-P Sol"=FALSE, "CryoP Pwr Relay 1"=FALSE, "CryoP Pwr Relay 2"=FALSE, "RoughP Pwr Relay"=FALSE}, "in"={"PG-SW-RoughP-Relay 1"=FALSE, "PG-SW-RoughP-Relay 2"=FALSE, "PG-SW-CryoP-Relay 1"=FALSE, "PG-SW-CryoP-Relay 2"=FALSE, "PG-SW-Chamber-Relay 1"=FALSE, "PG-SW-Chamber-Relay 2"=FALSE, "LN2-P-Sol-Open: NC"=FALSE, "LN2-P-Sol-Open: O"=FALSE, "LN2-P-Sol-Closed: NC"=FALSE, "LN2-P-Sol-Closed: O"=FALSE, "LN2-S-Sol-Open: NC"=FALSE, "LN2-S-Sol-Open: O"=FALSE, "LN2-S-Sol-Closed: NC"=FALSE, "LN2-S-Sol-Closed: O"=FALSE, "CryoP-GV-Open: NC"=FALSE, "CryoP-GV-Open: O"=FALSE, "CryoP-GV-Closed: NC"=FALSE, "CryoP-GV-Closed: O"=FALSE, "RoughP-GV-Open"=FALSE, "RoughP-GV-Closed"=FALSE, "RoughP-Pwr: NC"=FALSE, "RoughP-Pwr: O"=FALSE, "RoughP-On: NC"=FALSE, "RoughP-On: O"=FALSE, "Air supply LN2 OK"=FALSE, "Air supply OK"=FALSE}}) -> (value=w392:cluster{"out":T3, "in":T2})  [unwired: 5 in, 1 out]
        n183 = Unbundle By Name(w392) -> ("out"=w395:T3, "in"=→"Digi_In_1":T2)
        n184 = Bundle By Name(cluster=w397, "Http session"=w405) -> (w398:T6)
        n185 = local write "Digi_Out"(w395) -> ()
      }
      frame "GetPressure" {
        n186 = Unbundle By Name(w416) -> ("Http session"=w415:T5, "URL prefex"=w413:string)
        n187 = Build Array(3, 2, 1) -> (w411:i32[])
        n188 = Flatten To JSON(anything=w411) -> (JSON string=w410:string)  [unwired: 2 in, 1 out]
        n189 = Concatenate Strings(w413, "Pgauge" ("url")) -> (w414:string)
        n190 = call-poly <vilib>:"POST.vi"("client handle"=w415, "url"=w414, "buffer"=w410, "error in (no error)"=w420) -> ("client handle out"=w417:T5, "body"=w409:string, "error out"=w419:errorcluster)  [unwired: 8 in, 1 out]
        n191 = case shown="Default" w409 {
          selector: w409 -> [_ w434 w438]
          frame "" {
          }
          frame Default {
            n192 = Get Date/Time In Seconds() -> (seconds since 1Jan1904=w433:timestamp)
            n193 = Bundle By Name("t0"=w433) -> (w426:waveform(dbl))  [unwired: 1 in]
            n194 = Unflatten From JSON(JSON string=w434, type and defaults=T7 {"Addr"=[], "Kind"=[], "Pressure"=[], "Sw1 SP"=[], "Sw2 SP"=[]}) -> (value=w436:T7)  [unwired: 5 in, 1 out]
            n195 = Unbundle By Name(w436) -> ("Pressure"=w437:dbl[])
            n196 = Array To Cluster(array=w437) -> (cluster=w421:T13)
            "x/y" <- w421
            n197 = Unbundle(w421) -> ("Pressure[0]"=w432:dbl, "Pressure[1]"=w430:dbl, "Pressure[2]"=w431:dbl)
            n198 = Build Array(w432) -> (w427:dbl[])
            n199 = Build Array(w431) -> (w429:dbl[])
            n200 = Build Array(w430) -> (w428:dbl[])
            n201 = Bundle By Name(cluster=w426, "Y"=w427) -> (w425:waveform(dbl))
            n202 = Bundle By Name(cluster=w426, "Y"=w428) -> (w424:waveform(dbl))
            n203 = Bundle By Name(cluster=w426, "Y"=w429) -> (w423:waveform(dbl))
            n204 = Build Array(w425, w424, w423) -> (→"Waveform Chart":waveform(dbl)[])
          }
          frame "Buffer Needs to be list" {
            n205 = One Button Dialog(message=w438) -> ()  [unwired: 1 in, 1 out]
          }
        }
        n206 = Bundle By Name(cluster=w416, "Http session"=w417) -> (w418:T6)
      }
      frame "GetMCCstats" {
        n207 = Bundle("event"="get", "event"="Status", "event"="") -> (w444:T12)  [unwired: 1 in]
        n208 = Flatten To String(anything=w444) -> (data string=w445:string)  [unwired: 3 in, 2 out]
        n209 = call-poly "Send Message.vi"("error in (no error)"=w440, "event buffer"=w445, "event"="SendMCCcmd") -> ("error out"=w439:errorcluster)  [unwired: 8 in]
      }
      frame "MCC_GetParamValues" {
        n210 = Bundle("event"="get", "event"="ParamValues", "event"="") -> (w453:T12)  [unwired: 1 in]
        n211 = Flatten To String(anything=w453) -> (data string=w454:string)  [unwired: 3 in, 2 out]
        n212 = call-poly "Send Message.vi"("error in (no error)"=w449, "event buffer"=w454, "event"="SendMCCcmd") -> ("error out"=w448:errorcluster)  [unwired: 8 in]
      }
      frame "SendMCCcmd" {
        n213 = Unbundle By Name(w471) -> ("Http session"=w470:T5, "URL prefex"=w468:string)
        n214 = Unflatten From String(type=cluster{string, string, string} {"", "", ""}, binary string=w465) -> (value=w463:cluster{string, string, string})  [unwired: 3 in, 2 out]
        n215 = Unbundle(w463) -> (w457:string, w458:string, w461:string)
        n216 = Concatenate Strings(w468, "MCC_cmd/" ("url"), w457, "/" ("string"), w458) -> (w469:string)
        n217 = call-poly <vilib>:"POST.vi"("client handle"=w470, "url"=w469, "buffer"=w461, "error in (no error)"=w474) -> ("client handle out"=w472:T5, "body"=w466:string, "error out"=w460:errorcluster)  [unwired: 8 in, 1 out]
        n218 = case shown="Default" w466 {
          selector: w466 -> [_ w486]
          tunnel: w460 -> [w475 w482]
          tunnel: [w475 w481] -> w459
          tunnel: w458 -> [_ w480]
          tunnel: w457 -> [_ w478]
          frame "" {
          }
          frame Default {
            n219 = Unflatten From JSON(JSON string=w486, type and defaults=T8 {"Error"=FALSE, "PowerFailure"=FALSE, "Data"=""}) -> (value=w485:T8)  [unwired: 5 in, 1 out]
            n220 = Unbundle(w485) -> ("Error"=→"MCC Error":bool, "PowerFailure"=→"MCC Pwr":bool, "Data"=w479:string)
            "Resp" <- w479
            n221 = Concatenate Strings("MCC_" ("string"), w480) -> (w477:string)
            n222 = case shown="\"get\"" w478 {
              tunnel: w482 -> [w488 w492]
              tunnel: [w488 w491] -> w481
              tunnel: w477 -> [_ w490]
              tunnel: w479 -> [_ w489]
              frame Default {
              }
              frame "get" {
                n223 = call-poly "Send Message.vi"("error in (no error)"=w492, "event buffer"=w489, "event"=w490) -> ("error out"=w491:errorcluster)  [unwired: 8 in]
              }
            }
          }
        }
        n224 = Bundle By Name(cluster=w471, "Http session"=w472) -> (w473:T6)
      }
      frame "MCC_Status" {
        n225 = Unflatten From JSON(JSON string=w502, type and defaults=T9 {"Status"="", "TcPressure"="", "TempStage1"="", "TempStage2"="", "Duty Cycle"="", "RegenStep"="", "RegenError"="", "CryoPumpRdyState"=""}) -> (value=w501:T9)  [unwired: 5 in, 1 out]
        n226 = Unbundle By Name(w501) -> ("Status"=→"MCC_Status":string, "TcPressure"=→"MCC_TCpres":string, "TempStage1"=→"1st stage Temp":string, "TempStage2"=→"MCC 2nd stage Temp":string, "Duty Cycle"=→"DutyCycle":string, "RegenStep"=→"MCC_RegenSeq":string, "RegenError"=→"MCC_RegenError":string, "CryoPumpRdyState"=→"MCC_PumpState":string)
      }
      frame "MCC_ParamValues" {
        n227 = Unflatten From JSON(JSON string=w529, type and defaults=T10 {"MCCVersion"="", "ElapsedTime"="", "FirstStageTempCTL"="", "PurgeValveState"="", "RegenCycles"="", "RegenParam_0"="", "RegenParam_1"="", "RegenParam_2"="", "RegenParam_3"="", "RegenParam_4"="", "RegenParam_5"="", "RegenParam_6"="", "RegenParam_A"="", "RegenParam_C"="", "RegenParam_G"="", "RegenParam_z"="", "RegenTime"="", "RoughingValveState"="", "RoughingInterlock"="", "SecondStageTempCTL"="", "TcPressureState"=""}) -> (value=w527:T10)  [unwired: 5 in, 1 out]
        n228 = Unbundle By Name(w527) -> ("MCCVersion"=→"MCCget_Ver_V":string, "ElapsedTime"=→"CryoP OP Time":string, "FirstStageTempCTL"=→"MCC_1sgTempCtll V":string, "PurgeValveState"=→"MCC_TurnPurgeOn_V":string, "RegenCycles"=→"MCC_RegenCycles":string, "RegenParam_0"=→"Regen Restart Delay":string, "RegenParam_1"=→"Regen Ext Purge Time":string, "RegenParam_2"=→"Regen Repurge Cycles":string, "RegenParam_3"=→"Regen Rough to Press":string, "RegenParam_4"=→"Regen Rate of Rise":string, "RegenParam_5"=→"Regen Rt of Rise Cycles":string, "RegenParam_6"=→"Regen Restart Temp":string, "RegenParam_A"=→"Regen Rough Interlock":string, "RegenParam_C"=→"Pumps per Compressor":string, "RegenParam_G"=→"Regen Repurge Time":string, "RegenParam_z"=→"Regen Standby Mode":string, "RegenTime"=→"MCC_RegenTime":string, "RoughingValveState"=→"MCC_TurnRoughOn_V":string, "RoughingInterlock"=→"MCC_RoughInterlock_V":string, "SecondStageTempCTL"=→"MCC_2sgTempCtl V":string, "TcPressureState"=→"MCC_TurnTcOn_V":string)
      }
      frame "exit" {
        n229 = Unbundle By Name(w532) -> ("Http session"=w533:T5)
        n230 = Bundle By Name(cluster=w532, "go"=FALSE ("Bundle Element")) -> (w537:T6)
        n231 = call <vilib>:"CloseHandle.vi"("client handle"=w533, "error in (no error)"=w535) -> ("error out"=w534:errorcluster)  [unwired: 13 in]
      }
      frame Default {
        n232 = call "Unknown Message Dialog.vi"("source"=w539, "error in (no error)"=w541, "event name"=w540) -> ("error out"=w538:errorcluster)  [unwired: 8 in]
      }
    }
    n233 = Unbundle By Name(w12) -> ("go"=w11:bool)
    n234 = call "log system event.vi"("error in (no error)"=w9) -> ("error out"=w10:errorcluster)  [unwired: 9 in, 1 out]
  }
  n235 = call "Unload Module.vi"("error in (no error)"=w7) -> ()  [unwired: 10 in, 1 out]
